vi "AM Modulation Demo (Baseband-Music) - Template.vi"() -> ()   [LabVIEW 2013]
uses:
  <vilib>/sound2/lvsound2.llb/Sound File Info (path).vi
  <vilib>/sound2/lvsound2.llb/Sound File Read Open.vi
  <vilib>/sound2/lvsound2.llb/Sound File Read (DBL).vi
  <vilib>/Waveform/WDTOps.llb/WDT Get Waveform Subset DBL.vi
  <vilib>/express/express analysis/Spectral/Block/exnSpectralBlock spectral measurements RMS poly.vi
  <vilib>/express/express analysis/Spectral/Block/exnSpectralBlock spectral measurements RMS DDT.vi
  <vilib>/express/express analysis/Spectral/XNode/ExpressSpectralMeasurementsBlockNode.xnode
panel:
  in  "Path":path
  in  "Duration":dbl
  in  "WAV Sample Rate":dbl=44100.0 caption="dt"
  in  "Resample Rate":dbl=2000.0 caption="Frequency"
  in  "LPF Cut-Off":dbl=10000.0 caption="Lower Cut-Off"
  in  "AWGN (dB)":dbl(slide)=0.6 caption="Standard deviation" scale=-20.0..30.0
  out "Recovered Signal":dynamicdata(graph)
  out "Baseband":dynamicdata(graph)
  out "AM Wave FFT":dynamicdata(graph)
  out "AM Wave":dynamicdata(graph)
  in  "DC Offset":dbl=1.0
  in  "Carrier Amp.":dbl=1.0 caption="Amplitude"
  in  "stop":bool
  in  "Modulation Index":dbl(slide)=1.0 scale=0.0..5.0
  in  "Carrier Freq.":dbl=100000.0 caption="Frequency"
  out "After Rectifier":dynamicdata(graph)=[{"t0"=timestamp(0 s since 1904-01-01), "dt"=10.0, "Y"=array[50000 elements], "attributes"=variant("NI_ChannelName"=variant(string "Sine (Power Spectrum)"), "NI_ExpIsRelativeTime"=variant(bool TRUE), "NI_ExpStartTimeStamp"=variant(timestamp timestamp(3635665779.2842293 s since 1904-01-01)), "NI_ExpTimeStamp"=variant(timestamp timestamp(3635665779.2842293 s since 1904-01-01)), "NI_ExpXDimension"=variant(string "f"), "NI_OriginalChannelName"=variant(string "Sine"))}]
  # "Amplitude Modulation"
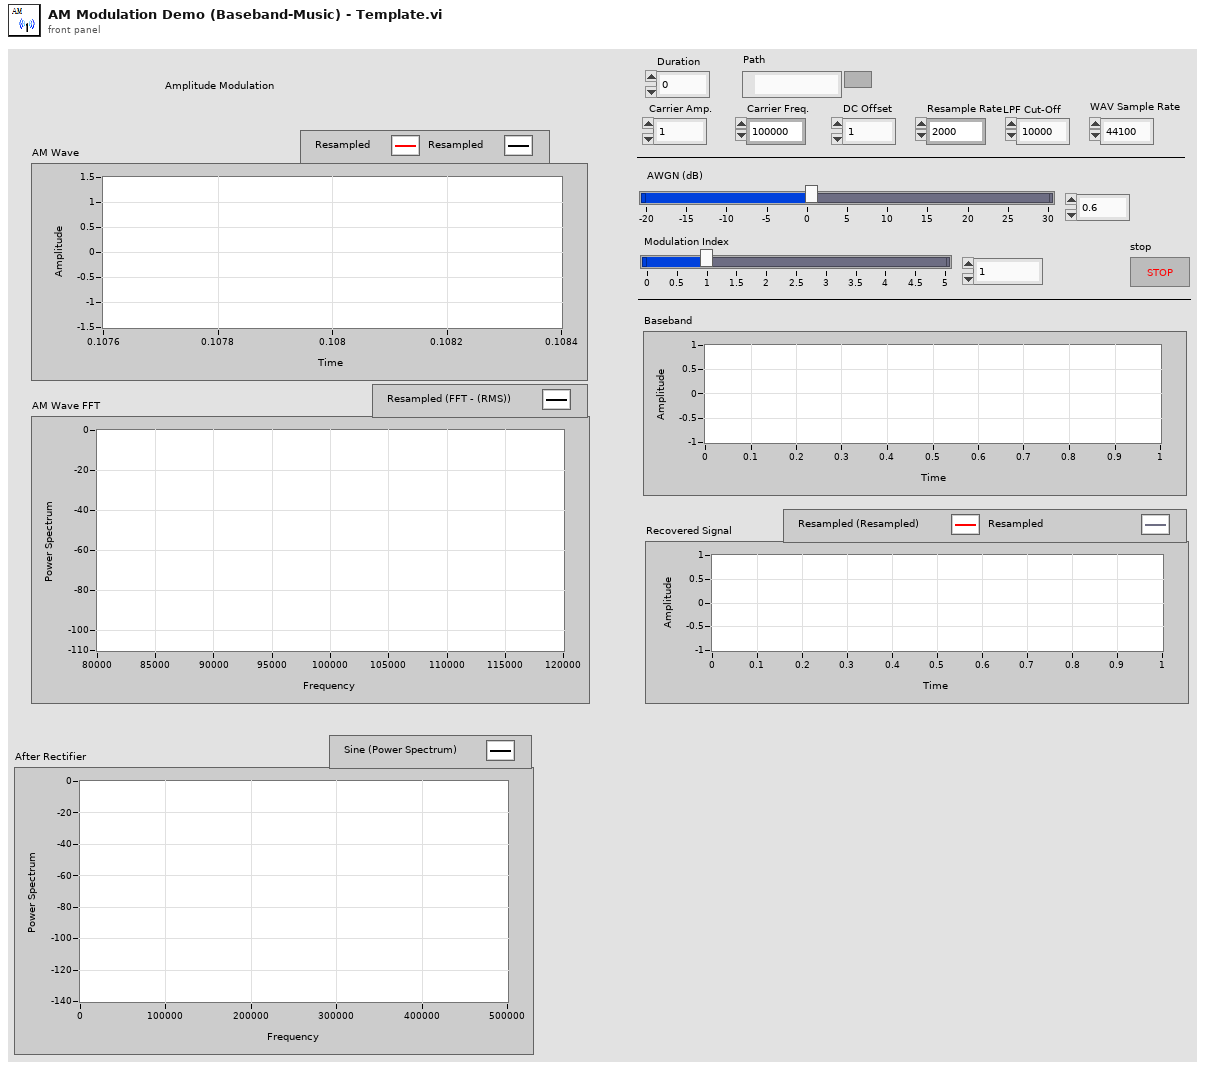
[diagram p1: front panel]
types:
  T1 = typedef "Sound File Refnum.ctl" = refnum<file>
  T2 = cluster{"averaging mode":u16, "weighting mode":u16, "number of averages":u32}
  T3 = cluster{"dB On (F)":bool, "unwrap phase (F)":bool, "convert to degree (F)":bool}
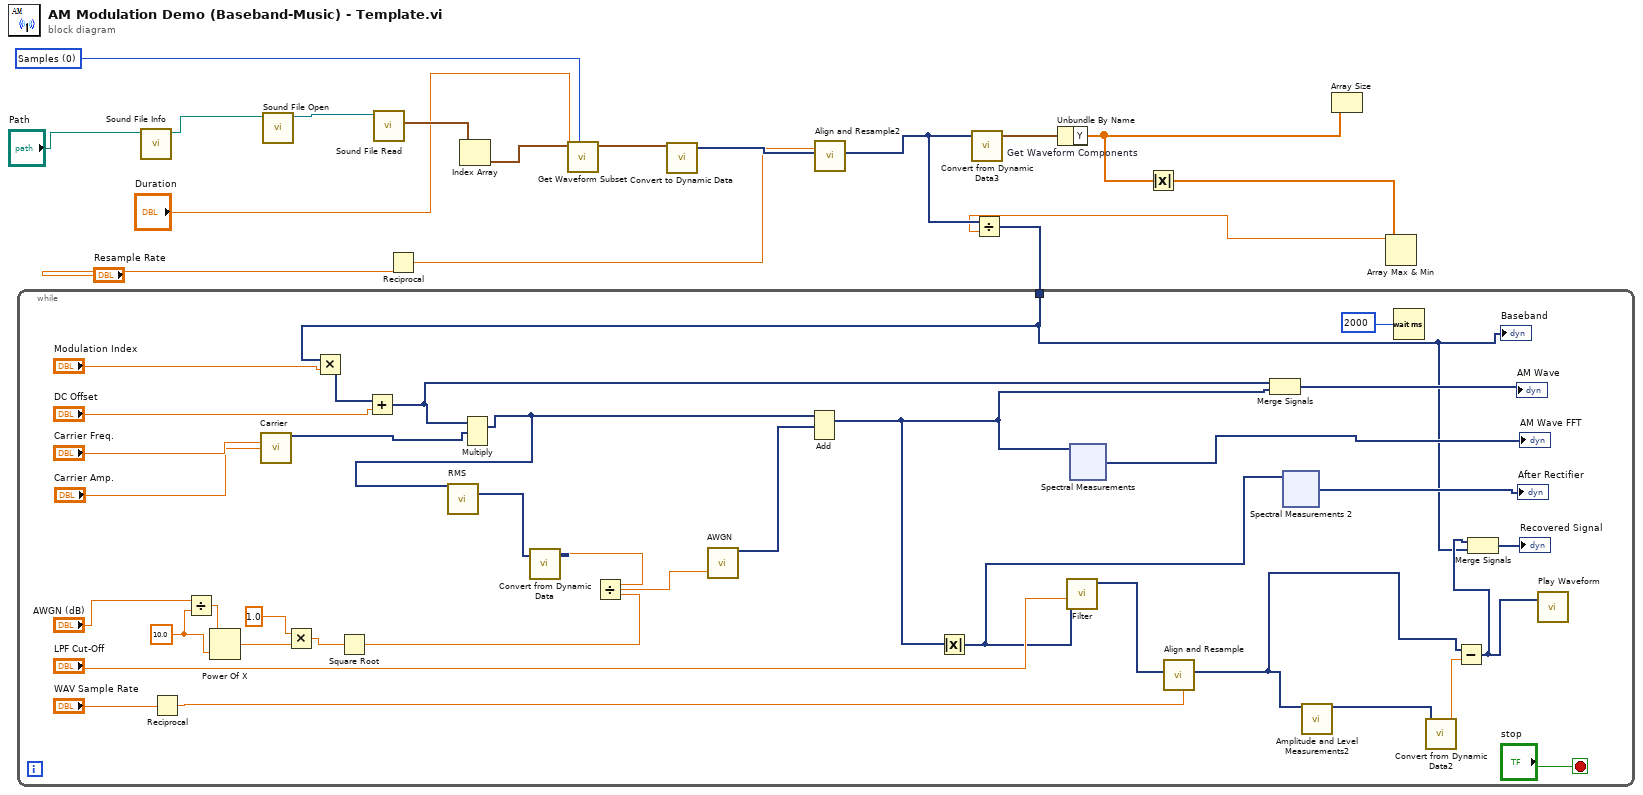
[diagram p0: block diagram]
diagram:
  w11 = u16 0 items=["Samples", "Relative Time"] ("start/duration format")
  n1 = call-poly <vilib>:"Sound File Info.vi"("path"="Path") -> ("path out"=w16:path)  [unwired: 7 in, 3 out]
  n2 = call-poly <vilib>:"Sound File Open.vi"("path"=w16) -> ("sound file refnum"=w15:T1)  [unwired: 9 in, 1 out]
  n3 = call-poly <vilib>:"Sound File Read.vi"("sound file refnum"=w15) -> ("data"=w14:waveform(dbl)[])  [unwired: 6 in, 4 out]
  n4 = Reciprocal(x="Resample Rate") -> (1/x=w8:dbl)
  n5 = Index Array "Index Array"(array=w14) -> (element=w13:waveform(dbl))  [unwired: 1 in]
  n6 = call-poly <vilib>:"Get Waveform Subset.vi"("start/duration format"=w11, "duration"="Duration", "waveform in"=w13) -> ("waveform out"=w1:waveform(dbl))  [unwired: 3 in, 3 out]
  n7 = call "Convert to Dynamic Data"("Waveform"=w1) -> ("Dynamic Data Type"=w10:dynamicdata)  [unwired: 3 in]
  n8 = call "Align and Resample2"("dt"=w8, "Signals"=w10) -> ("Resampled Signals"=w3:dynamicdata)  [unwired: 7 in, 2 out]
  n9 = call "Convert from Dynamic Data3"("Dynamic Data Type"=w3) -> ("Waveform"=w7:waveform(dbl))  [unwired: 3 in]
  n10 = Unbundle By Name "Get Waveform Components"(w7) -> ("Y"=w6:dbl[])
  n11 = Absolute Value(x=w6) -> (abs(x)=w5:dbl[])
  n12 = Array Size(array=w6) -> ()  [unwired: 1 out]
  n13 = Array Max & Min(array=w5) -> (max value=w2:dbl)  [unwired: 3 out]
  n14 = Divide(x=w3, y=w2) -> (x/y=w4:dynamicdata)
  n15 = while {
    tunnel: w4 -> [w18]
    stop <- "stop" stop-if-true
    w26 = 10.0
    n16 = Reciprocal(x="WAV Sample Rate") -> (1/x=w33:dbl)
    n17 = Divide(x="AWGN (dB)", y=w26) -> (x/y=w27:dbl)
    n18 = Power Of X(1:w26, 2:w27) -> (0:w25:dbl)
    n19 = call "Carrier"("Frequency"="Carrier Freq.", "Amplitude"="Carrier Amp.") -> ("Sine"=w47:dynamicdata)  [unwired: 12 in, 1 out]
    n20 = Multiply(x=1.0, y=w25) -> (x*y=w40:dbl)
    n21 = Multiply(x=w18, y="Modulation Index") -> (x*y=w51:dynamicdata)
    n22 = Square Root(x=w40) -> (sqrt(x)=w38:dbl)
    n23 = Add(x=w51, y="DC Offset") -> (x+y=w45:dynamicdata)
    n24 = Multiply(1:w47, 2:w45) -> (0:w37:dynamicdata)  [unwired: 1 in, 1 out]
    n25 = call "RMS"("Signals"=w37) -> ("RMS"=w44:dynamicdata)  [unwired: 13 in, 1 out]
    n26 = call "Convert from Dynamic Data"("Dynamic Data Type"=w44) -> ("Scalar"=w39:dbl)  [unwired: 3 in]
    n27 = Divide(x=w39, y=w38) -> (x/y=w24:dbl)
    n28 = call "AWGN"("Standard deviation"=w24) -> ("DC with Gaussian Noise"=w36:dynamicdata)  [unwired: 13 in, 1 out]
    n29 = Add(1:w36, 2:w37) -> (0:w34:dynamicdata)  [unwired: 1 in, 1 out]
    n30 = Absolute Value(x=w34) -> (abs(x)=w20:dynamicdata)
    n31 = call "Filter"("Lower Cut-Off"="LPF Cut-Off", "Signal"=w20) -> ("Filtered Signal"=w32:dynamicdata)  [unwired: 8 in, 1 out]
    n32 = xnode "Spectral Measurements"("Signals"=w34) -> ("FFT - (RMS)"=→"AM Wave FFT":dynamicdata)  [unwired: 1 in, 2 out]
    n33 = call "Align and Resample"("dt"=w33, "Signals"=w32) -> ("Resampled Signals"=w21:dynamicdata)  [unwired: 7 in, 2 out]
    n34 = Merge Signals(w45, w34) -> (→"AM Wave":dynamicdata)
    n35 = xnode "Spectral Measurements 2"("Signals"=w20) -> ("FFT - (RMS)"=→"After Rectifier":dynamicdata)  [unwired: 1 in, 2 out]
    n36 = call "Amplitude and Level Measurements2"("Signals"=w21) -> ("Mean (DC)"=w22:dynamicdata)  [unwired: 13 in, 1 out]
    n37 = Wait (ms)(milliseconds to wait=2000) -> ()  [unwired: 1 out]
    n38 = call "Convert from Dynamic Data2"("Dynamic Data Type"=w22) -> ("Scalar"=w29:dbl)  [unwired: 3 in]
    n39 = Subtract(x=w21, y=w29) -> (x-y=w23:dynamicdata)
    n40 = Merge Signals(w23, w18) -> (→"Recovered Signal":dynamicdata)
    n41 = call "Play Waveform"("Data"=w23) -> ()  [unwired: 18 in, 1 out]
    "Baseband" <- w18
  }
